vi "KLB Image Spaces.vi"(8 "error in (no error)":errorcluster, 11 "Reset?":bool) -> (0 "error out":errorcluster, 2 "RGB Image":T1, 3 "U8 Image":T1)   [LabVIEW 2013]
doc: "Creates a tempory RGB image space along with unique image spaces for all the KLB images."
uses:
  <vilib>/vision/Image Controls.llb/IMAQ Image.ctl
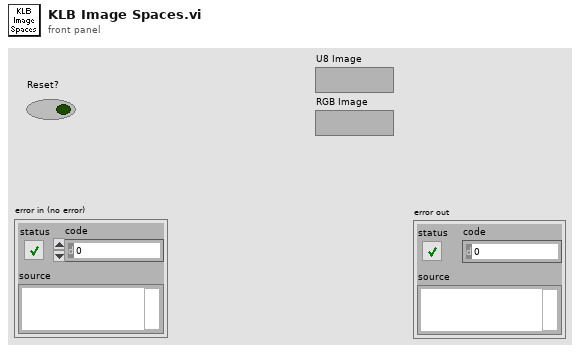
[diagram p1: front panel]
types:
  T1 = typedef "IMAQ Image.ctl" = refnum<image>
  T2 = typedef "Image Type" = u32
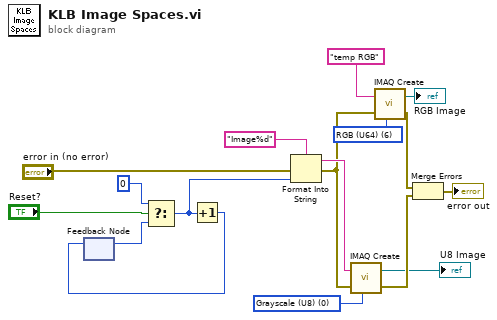
[diagram p0: block diagram]
diagram:
  w15 = T2 0 items=["Grayscale (U8)", "Grayscale (I16)", "Grayscale (SGL)", "Complex (CSG)", "RGB (U32)", "HSL (U32)", "RGB (U64)", "Grayscale (U16)"] ("Image Type")
  w16 = T2 6 items=["Grayscale (U8)", "Grayscale (I16)", "Grayscale (SGL)", "Complex (CSG)", "RGB (U32)", "HSL (U32)", "RGB (U64)", "Grayscale (U16)"] ("Image Type")
  n1 = feedback #1() -> (w8:i32)  [unwired: 1 in]
  n2 = Select(t=0 ("input 1"), s="Reset?", f=w8) -> (s? t:f=w6:i32)
  n3 = Increment(x=w6) -> (x+1=w7:i32)
  n4 = feedback-in #1(w7) -> ()
  n5 = Format Into String(format string="Image%d", error in="error in (no error)", w6) -> (resulting string=w14:string, error out=w13:errorcluster)  [unwired: 1 in]
  n6 = call "IMAQ Create"("Image Name"=w14, "Image Type"=w15, "error in (no error)"=w13) -> ("New Image"=→"U8 Image":T1, "error out"=w11:errorcluster)  [unwired: 2 in]
  n7 = call "IMAQ Create"("Image Name"="temp RGB", "Image Type"=w16, "error in (no error)"=w13) -> ("New Image"=→"RGB Image":T1, "error out"=w12:errorcluster)  [unwired: 2 in]
  n8 = Merge Errors(w12, w11) -> (→"error out":errorcluster)
